vi "Build Config File Absolute Path.vi"(0 "Sequence File Path":path, 11 "error in (no error)":errorcluster) -> (6 "Config File Absolute Path":path, 15 "error out":errorcluster)   [LabVIEW 2023, in "RFCalAndFixtureCharact.Common.lvlib"]
uses:
  RFCalAndFixtureCharact.Common.lvlib
  Data Cache/Settings Dictionary/Setting Keys.vi
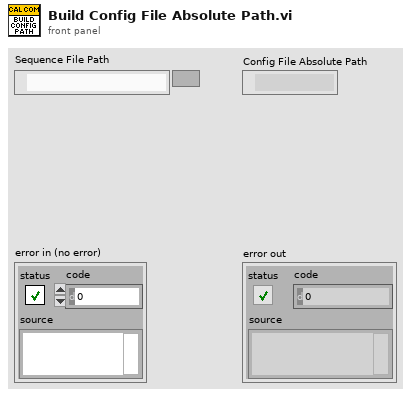
[diagram p1: front panel]
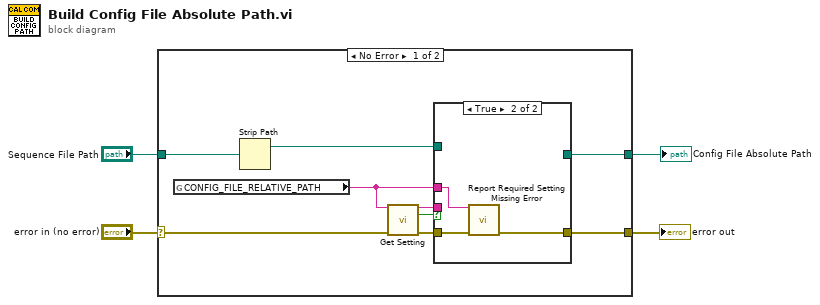
[diagram p0: block diagram]
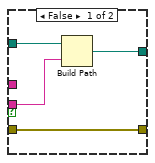
[diagram p2: hidden frame]
diagram:
  n1 = case shown="No Error" "error in (no error)" {
    selector: "error in (no error)" -> [w11 w21]
    tunnel: [w12 w21] -> w3
    tunnel: "Sequence File Path" -> [w6 _]
    tunnel: [w13 _] -> w1
    frame No Error {
      n2 = global read "Setting Keys.vi" "CONFIG_FILE_RELATIVE_PATH"() -> (w7:string)
      n3 = Strip Path(path=w6) -> (stripped path=w5:path)  [unwired: 1 out]
      n4 = call "Get Setting.vi"("Setting name"=w7, "error in (no error)"=w11) -> ("Setting value out"=w8:string, "Setting empty or not found?"=w9:bool, "error out"=w10:errorcluster)  [unwired: 11 in]
      n5 = case shown="True" w9 {
        tunnel: w5 -> [w17 _]
        tunnel: [w16 _] -> w13
        tunnel: [w15 w19] -> w12
        tunnel: w10 -> [w15 w20]
        tunnel: w8 -> [w14 _]
        tunnel: w7 -> [_ w18]
        frame False {
          n6 = Build Path(base path=w17, name or relative path=w14) -> (appended path=w16:path)
        }
        frame True {
          n7 = call "Report Required Setting Missing Error.vi"("Setting name"=w18, "Error in (no error)"=w20) -> ("error out"=w19:errorcluster)  [unwired: 13 in]
        }
      }
    }
    frame Error {
    }
  }
  "error out" <- w3
  "Config File Absolute Path" <- w1
